vi "Set Value and Output.vi"(5 "Enable Output (T: Enable)":bool=TRUE, 6 "error in (no error)":errorcluster, 7 "Voltage Level (0.0 V)":dbl caption="Voltage Level (0 V)" format="%.2f", 8 "CH number":i32, 9 "VISA resource name":refnum<visa-resource-name>) -> (0 "error out":errorcluster, 3 "VISA resource name out":refnum<visa-resource-name>)   [LabVIEW 2023, in "Rigol.lvlib"]
uses:
  Rigol.lvlib
  <instrlib>/RIGOL DP800 Series/Public/Channels.ctl
  <instrlib>/RIGOL DP800 Series/RIGOL DP800 Series.lvlib
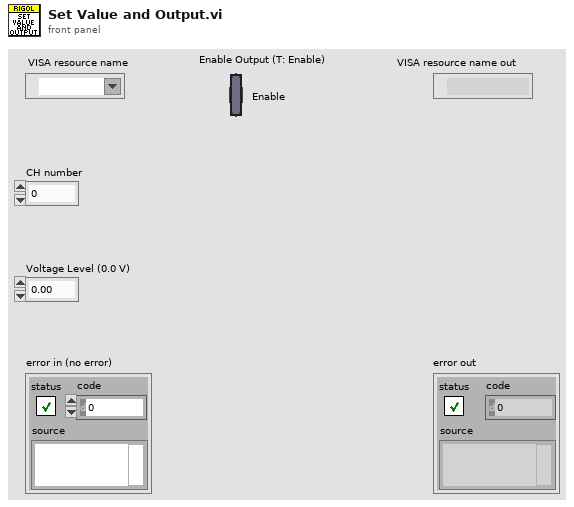
[diagram p1: front panel]
types:
  T1 = typedef "RIGOL DP800 Series.lvlib/Channels.ctl" = i32
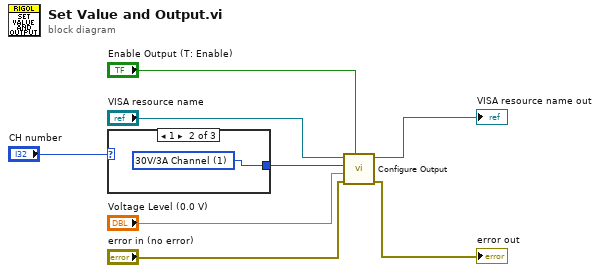
[diagram p0: block diagram]
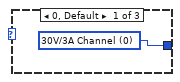
[diagram p2: hidden frame]
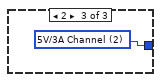
[diagram p3: hidden frame]
diagram:
  n1 = case shown="1" "CH number" {
    tunnel: [w9 w10 w11] -> w1
    frame 0, Default {
      w9 = T1 0 items=["30V/3A Channel", "30V/3A Channel", "5V/3A Channel"] ("Channel (0: 30V Channel)")
    }
    frame 1 {
      w10 = T1 1 items=["30V/3A Channel", "30V/3A Channel", "5V/3A Channel"] ("Channel (0: 30V Channel)")
    }
    frame 2 {
      w11 = T1 2 items=["30V/3A Channel", "30V/3A Channel", "5V/3A Channel"] ("Channel (0: 30V Channel)")
    }
  }
  n2 = call <instrlib>:"Configure Output.vi"("Enable Output (T: Enable)"="Enable Output (T: Enable)", "error in (no error)"="error in (no error)", "Voltage Level (0.0 V)"="Voltage Level (0.0 V)", "Channel (0: 30V Channel)"=w1, "VISA resource name"="VISA resource name") -> ("error out"=→"error out":errorcluster, "VISA resource name out"=→"VISA resource name out":refnum<visa-resource-name>)  [unwired: 5 in]
